vi "Stable_1Parameter.vi"(0 "VISA resource name":refnum<visa-resource-name>, 5 "Parameter (1: X)":u16(ring)=1 items=["X"=1, "Y"=2, "R"=3, "Theta"=4, "Channel 1"=5, "Channel 2"=6, "Aux In 1"=7, "Aux In 2"=8, "Aux In 3"=9, "Aux In 4"=10], 9 "Max loop n":i32=20, 11 "milliseconds to wait":u32=150, 12 "error in (no error)":errorcluster) -> (4 "VISA resource name out":refnum<visa-resource-name>, 6 "1 parameter (final mean)":dbl, 15 "error out":errorcluster)   [LabVIEW 2017]
uses:
  Program Files (x86)/National Instruments/LabVIEW 2017/instr.lib/Stanford Research 830/Public/Data/Read (1 Parameter).vi
  Documents/Data/Chunxiong Bao/Capacitance/SR830/Stanford Research 830/Stanford Research 830.lvlib
panel:
  out "Numeric 3":dbl
  out "Numeric 2":dbl
  out "Numeric":dbl
  out "Average":dbl[](array[numeric])
  out "3 latest R values":dbl[](array[numeric])
  out "All Lock-in R values":dbl[](array[numeric])
  out "Loop ued":i32
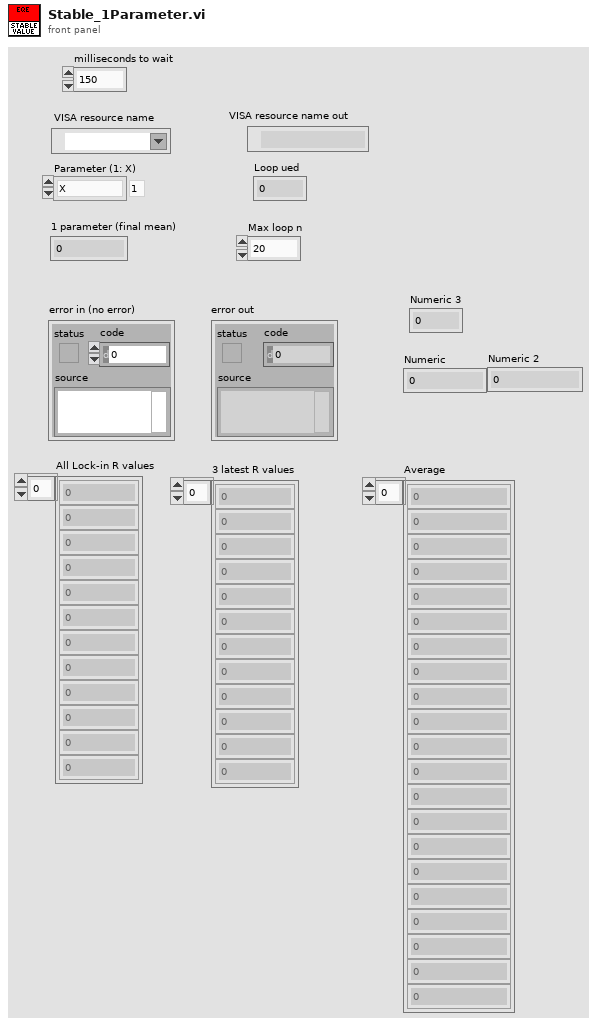
[diagram p1: front panel]
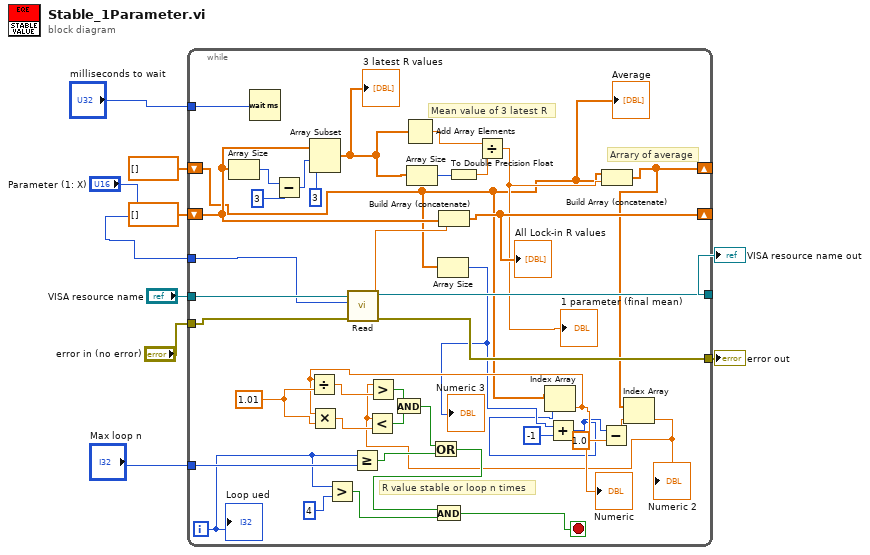
[diagram p0: block diagram]
diagram:
  n1 = while {
    tunnel: "VISA resource name" -> [w49]
    tunnel: "error in (no error)" -> [w48]
    shift-right: [w43] -> _
    shift-left: dbl[] [] -> [w34]
    tunnel: "Parameter (1: X)" -> [w30]
    tunnel: [w29] -> w7
    tunnel: [w28] -> w6
    tunnel: "Max loop n" -> [w27]
    tunnel: "milliseconds to wait" -> [w26]
    shift-right: [w11] -> _
    shift-left: dbl[] [] -> [w12]
    i -> [w25]
    stop <- w21 stop-if-true
    w38 = 1.01 ("y")
    # "Arrary of average"
    # "Mean value of 3 latest R"
    # "R value stable or loop n times"
    n2 = Array Size(array=w34) -> (size(s)=w20:i32)
    n3 = Wait (ms)(milliseconds to wait=w26) -> ()  [unwired: 1 out]
    n4 = Subtract(x=w20, y=3) -> (x-y=w32:i32)
    n5 = Array Subset(array=w34, index=w32, length=3) -> (w31:dbl[])
    "3 latest R values" <- w31
    n6 = Greater?(x=w25, y=4) -> (0:w23:bool)
    n7 = call-poly "Read.vi"("error in (no error)"=w48, "Parameter (1: X)"=w30, "VISA resource name"=w49) -> ("error out"=w29:errorcluster, "Measurement"=w39:dbl, "VISA resource name out"=w28:refnum<visa-resource-name>)  [unwired: 6 in]
    n8 = Greater Or Equal?(x=w25, y=w27) -> (x >= y?=w47:bool)
    n9 = Add Array Elements(numeric array=w31) -> (sum=w44:dbl)
    n10 = Array Size(array=w31) -> (size(s)=w46:i32)
    n11 = Array Size(array=w12) -> (size(s)=w16:i32)
    "Numeric 3" <- w16
    n12 = Build Array (concatenate)(w34, w39) -> (w43:dbl[])
    "All Lock-in R values" <- w43
    n13 = To Double Precision Float(number=w46) -> (double precision float=w45:dbl)
    n14 = Divide(x=w44, y=w45) -> (x/y=w17:dbl)
    "1 parameter (final mean)" <- w17
    n15 = Add(x=w16, y=-1) -> (x+y=w13:i32)
    n16 = Index Array(array=w12, index=w13) -> (element=w18:dbl)
    "Numeric" <- w18
    n17 = Divide(x=w18, y=w38) -> (x/y=w37:dbl)
    n18 = Multiply(x=w18, y=w38) -> (x*y=w36:dbl)
    n19 = Subtract(x=w13, y=1.0) -> (x-y=w14:dbl)
    n20 = Build Array (concatenate)(w12, w17) -> (w11:dbl[])
    n21 = Index Array(array=w11, index=w14) -> (element=w10:dbl)
    "Numeric 2" <- w10
    n22 = Less?(x=w10, y=w36) -> (x < y?=w42:bool)
    n23 = Greater?(x=w10, y=w37) -> (0:w41:bool)
    n24 = And(x=w41, y=w42) -> (x .and. y?=w40:bool)
    n25 = Or(x=w40, y=w47) -> (x .or. y?=w22:bool)
    n26 = And(x=w22, y=w23) -> (x .and. y?=w21:bool)
    "Loop ued" <- w25
    "Average" <- w12
  }
  "error out" <- w7
  "VISA resource name out" <- w6
